vi "Named ROIs to ROI Descriptors.vi"(11 "Named ROIs":T1[](array[typedef]) {"ROI Descriptor"."Contours"."Type" items=["No Selection", "Point", "Line", "Rectangle", "Oval", "Polygon", "Freehand Region", "Annulus", "Unused2", "Unused3", "Broken Line", "Freehand Line", "Rotated Rectangle"]}) -> (3 "ROI Descriptors":T2[](array[typedef]) {"Contours"."Type" items=["No Selection", "Point", "Line", "Rectangle", "Oval", "Polygon", "Freehand Region", "Annulus", "Unused2", "Unused3", "Broken Line", "Freehand Line", "Rotated Rectangle"]})   [LabVIEW 2021, in "Image.lvlib"]
uses:
  Image.lvlib
  Named ROI Description.ctl
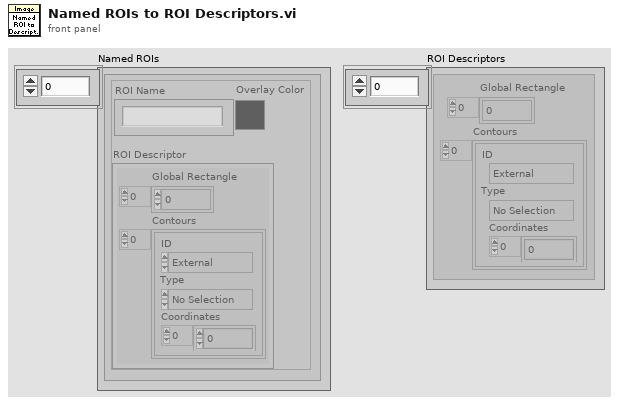
[diagram p1: front panel]
types:
  T1 = typedef "Image.lvlib/Named ROI Description.ctl" = cluster{"ROI Descriptor":T2, "ROI Name":string, "Overlay Color":u32}
  T2 = typedef "ROI Descriptor" = cluster{"Global Rectangle":i32[], "Contours":cluster{"ID":enum32{"External", "Internal"}, "Type":u32, "Coordinates":i32[]}[]}
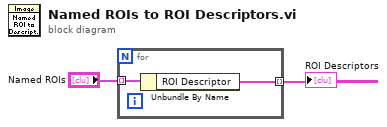
[diagram p0: block diagram]
diagram:
  n1 = for {
    tunnel: "Named ROIs" -> [w4] mode=indexing
    tunnel: [w3] -> w1 mode=indexing
    n2 = Unbundle By Name(w4) -> ("ROI Descriptor"=w3:T2)
  }
  "ROI Descriptors" <- w1
